vi "Kill all AMC Queues.vi"   [LabVIEW 2011]
doc: "Kills all AMC queues that are still running.\n\n\nVersion 1.0 - 02/13/2013\n\nPhaeron, Inc.\nwww.phaeron.com\ninfo@phaeron.com"
uses:
  <vilib>/NI/AMC/AMC.lvlib
types:
  T1 = typedef "AMC.lvlib/Message Queue.ctl" = refnum<queue>
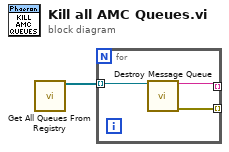
[diagram p0: block diagram]
diagram:
  n1 = call <vilib>:"Get All Queues From Registry.vi"() -> ("all queues"=w1:T1[])  [unwired: 12 in, 3 out]
  n2 = for {
    tunnel: w1 -> [w4] mode=indexing
    tunnel: [w3] -> _ mode=indexing
    tunnel: [w2] -> _ mode=indexing
    n3 = call <vilib>:"Destroy Message Queue.vi"("message queue in"=w4) -> ("message queue name"=w2:string, "error out"=w3:errorcluster)  [unwired: 12 in, 1 out]
  }
